vi "Test Slack XControl.vi"() -> ()   [LabVIEW 2015]
uses:
  Slack/Slack.xctl
  Typedefs/Slack-Configuration.ctl
  Typedefs/Slack-User.ctl
panel:
  out "users":T1[](array[typedef])
  out "config":T2
  in  "Slack":cluster{"config":T2, "users":T1[]}(xcontrol)
  in  "stop":bool
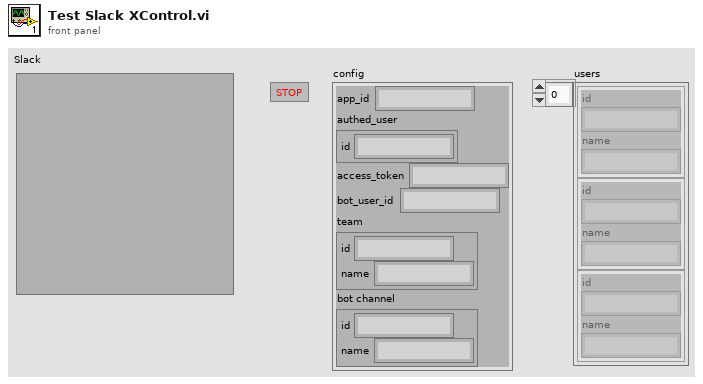
[diagram p1: front panel]
types:
  T1 = typedef "Slack-User.ctl" = cluster{"id":string, "name":string}
  T2 = typedef "Slack-Configuration.ctl" = cluster{"app_id":string, "authed_user":cluster{"id":string}, "access_token":string, "bot_user_id":string, "team":cluster{"id":string, "name":string}, "bot channel":cluster{"id":string, "name":string}}
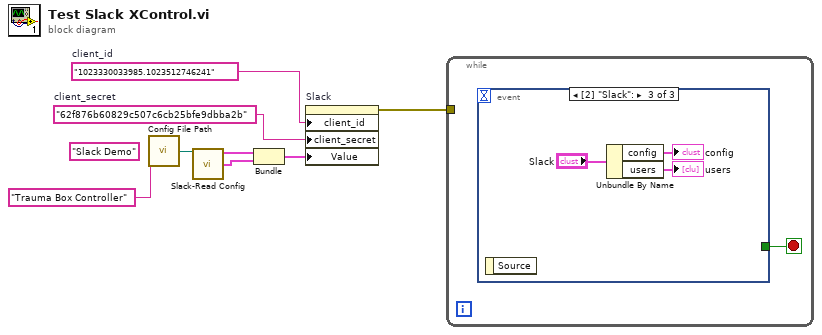
[diagram p0: block diagram]
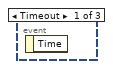
[diagram p2: hidden frame]
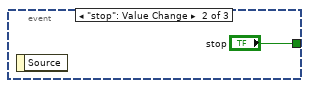
[diagram p3: hidden frame]
diagram:
  w4 = "62f876b60829c507c6cb25bfe9dbba2b"  # client_secret
  w5 = "1023330033985.1023512746241"  # client_id
  (unwired) "Slack Demo" ("AppName")
  n1 = call "Config File Path.vi"("AppName"="Trauma Box Controller") -> ("Default config file name"=w8:path)
  n2 = call "Slack-Read Config.vi"("AppName"=w8) -> ("config"=w7:T2, "users"=w6:T1[])  [unwired: 12 in, 1 out]
  n3 = Bundle("config"=w7, "users"=w6) -> (w3:cluster{"config":T2, "users":T1[]})  [unwired: 1 in]
  n4 = property on="Slack" class="Slack (strict)"("client_id"=w5, "client_secret"=w4, "Value"=w3) -> (error out=w2:errorcluster)  [unwired: 2 in, 1 out]
  n5 = while {
    tunnel: w2 -> [_]
    stop <- w9 stop-if-true
    n6 = event shown="[2] \"Slack\":" {
      selector: _ -> [_ _ _]
      dyn-events: _ -> [_ _ _]
      timeout: _ -> [_ _ _]
      tunnel: [_ "stop" _] -> w9
      event Timeout {
        n7 = event-data() -> ()  [unwired: 1 in, 1 out]
      }
      event "stop": Value Change {
        n8 = event-data() -> ()  [unwired: 1 in, 1 out]
      }
      event "Slack": Value Change {
        n9 = event-data() -> ()  [unwired: 1 in, 1 out]
        n10 = Unbundle By Name("Slack") -> ("config"=→"config":T2, "users"=→"users":T1[])
      }
    }
  }
